vi "MaxDisplay.vi"(0 "VisaCluster":T2, 7 "Max":T1, 11 "error in (no error)":errorcluster) -> (4 "VisaCluster 2":T2, 6 "Answer":string, 8 "Max 2":T1, 15 "error out":errorcluster)   [LabVIEW 2014, in "FH 55.lvlib"]
doc: "Dieses VI wird aktuell nicht genutzt. Es liest die Extremwerte direkt aus dem Gerät. Die Extremwerte werden durch MaxFunktion ermittelt"
uses:
  FH 55.lvlib
  TypeDef/Max.ctl
  TypeDef/VisaCluster.ctl
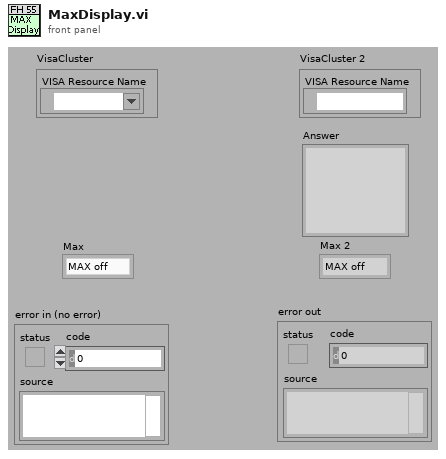
[diagram p1: front panel]
types:
  T1 = typedef "FH 55.lvlib/Max.ctl" = enum16{"MAX off", "Show MAX", "MAX/MIN"}
  T2 = typedef "FH 55.lvlib/VisaCluster.ctl" = cluster{"VISA Resource Name":refnum<visa-resource-name>}
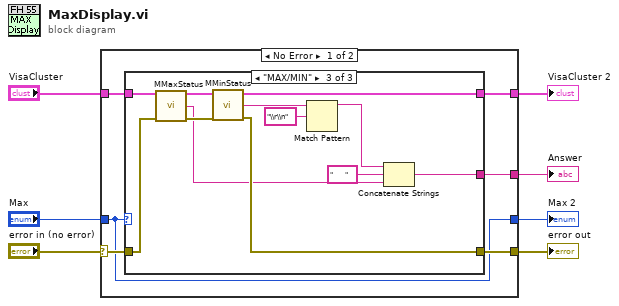
[diagram p0: block diagram]
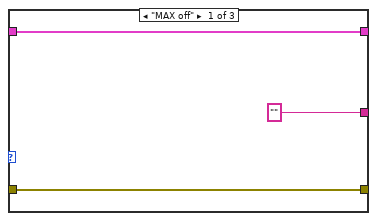
[diagram p2: hidden frame]
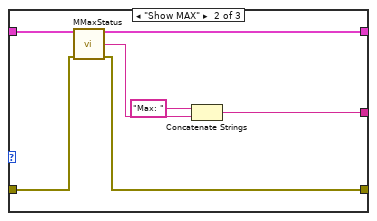
[diagram p3: hidden frame]
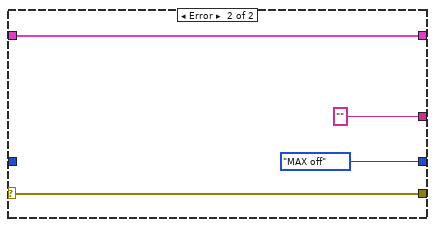
[diagram p4: hidden frame]
diagram:
  n1 = case shown="No Error" "error in (no error)" {
    selector: "error in (no error)" -> [w11 w38]
    tunnel: [w8 Max."MAX off" ("Max 2")] -> w7
    tunnel: [w13 "" ("Answer")] -> w6
    tunnel: "VisaCluster" -> [w12 w39]
    tunnel: "Max" -> [w8 _]
    tunnel: [w9 w39] -> w3
    tunnel: [w10 w38] -> w2
    frame No Error {
      n2 = case shown="\"MAX/MIN\"" w8 {
        tunnel: w12 -> [w14 w23 w35]
        tunnel: ["" w17 w31] -> w13
        tunnel: w11 -> [w15 w22 w30]
        tunnel: [w15 w21 w29] -> w10
        tunnel: [w14 w20 w28] -> w9
        frame "MAX off" {
        }
        frame "Show MAX" {
          n3 = call "MMaxStatus.vi"("VisaCluster"=w23, "error in (no error)"=w22) -> ("VisaCluster"=w20:T2, "Answer"=w18:string, "error out"=w21:errorcluster)  [unwired: 11 in]
          n4 = Concatenate Strings("Max: " ("string"), w18) -> (w17:string)
        }
        frame "MAX/MIN" {
          n5 = call "MMaxStatus.vi"("VisaCluster"=w35, "error in (no error)"=w30) -> ("VisaCluster"=w34:T2, "Answer"=w27:string, "error out"=w33:errorcluster)  [unwired: 11 in]
          n6 = call "MMinStatus.vi"("VisaCluster"=w34, "error in (no error)"=w33) -> ("VisaCluster"=w28:T2, "Answer"=w25:string, "error out"=w29:errorcluster)  [unwired: 11 in]
          n7 = Match Pattern(string=w25, regular expression="\\r\\n") -> (before substring=w24:string)  [unwired: 1 in, 3 out]
          n8 = Concatenate Strings(w24, "      " ("string"), w27) -> (w31:string)
        }
      }
    }
    frame Error {
    }
  }
  "Max 2" <- w7
  "Answer" <- w6
  "error out" <- w2
  "VisaCluster 2" <- w3
